vi "put into robot.vi"(8 "error in (no error)":errorcluster) -> (0 "error out":errorcluster)   [LabVIEW 2019]
uses:
  servo state.ctl
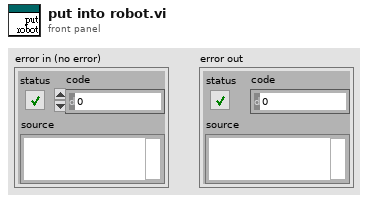
[diagram p1: front panel]
types:
  T1 = typedef "servo state.ctl" = enum16{"catch", "cam-1", "put", "side", "center", "side-2"}
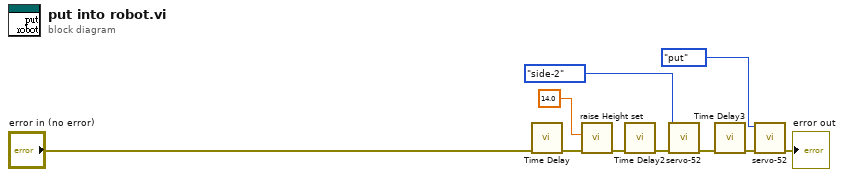
[diagram p0: block diagram]
diagram:
  n1 = call "Time Delay"("error in (no error)"="error in (no error)") -> ("error out"=w2:errorcluster)  [unwired: 10 in]
  n2 = call "raise Height set.vi"("error in (no error)"=w2, "Height_cm"=14.0) -> ("error out"=w5:errorcluster)  [unwired: 9 in]
  n3 = call "Time Delay2"("error in (no error)"=w5) -> ("error out"=w6:errorcluster)  [unwired: 10 in]
  n4 = call "servo-52.vi"("error in (no error)"=w6, "Enum"=servo_state."side-2") -> ("error out"=w7:errorcluster)  [unwired: 9 in]
  n5 = call "Time Delay3"("error in (no error)"=w7) -> ("error out"=w9:errorcluster)  [unwired: 10 in]
  n6 = call "servo-52.vi"("error in (no error)"=w9, "Enum"=servo_state."put") -> ("error out"=→"error out":errorcluster)  [unwired: 9 in]
